vi "fit_characteristics.vi"(10 "Polynomial Coefficients":dbl[][](array[numeric]), 11 "Residue":dbl[](array[numeric])) -> (1 "Limit fail":bool[][](array[boolean]), 3 "Fit characteristics":string[][](table))   [LabVIEW 2013]
uses:
  <vilib>/Analysis/polynomials.llb/nth Derivative of Polynomial (DBL).vi
  <vilib>/Analysis/polynomials.llb/Scalar Polynomial Evaluation (DBL).vi
  <vilib>/Analysis/polynomials.llb/1D Polynomial Evaluation (DBL).vi
  <vilib>/Analysis/NI_AALPro.lvlib
panel:
  out "All x":dbl[][](array[numeric])
  out "Labels":string[](array[string])
  in  "Limits":cluster{"Min":dbl, "Max":dbl}[](array[cluster])=[{"Min"=2.0, "Max"=inf}, {"Min"=0.0, "Max"=0.3}, {"Min"=10.0, "Max"=inf}, {"Min"=10.0, "Max"=inf}, {"Min"=-inf, "Max"=-10.0}, {"Min"=10.0, "Max"=inf}, {"Min"=0.0, "Max"=1.0}]
  # "True if the corresponding  cell of the table should be highlighted as as failing limit test."
  # "Generate report of calibration results."
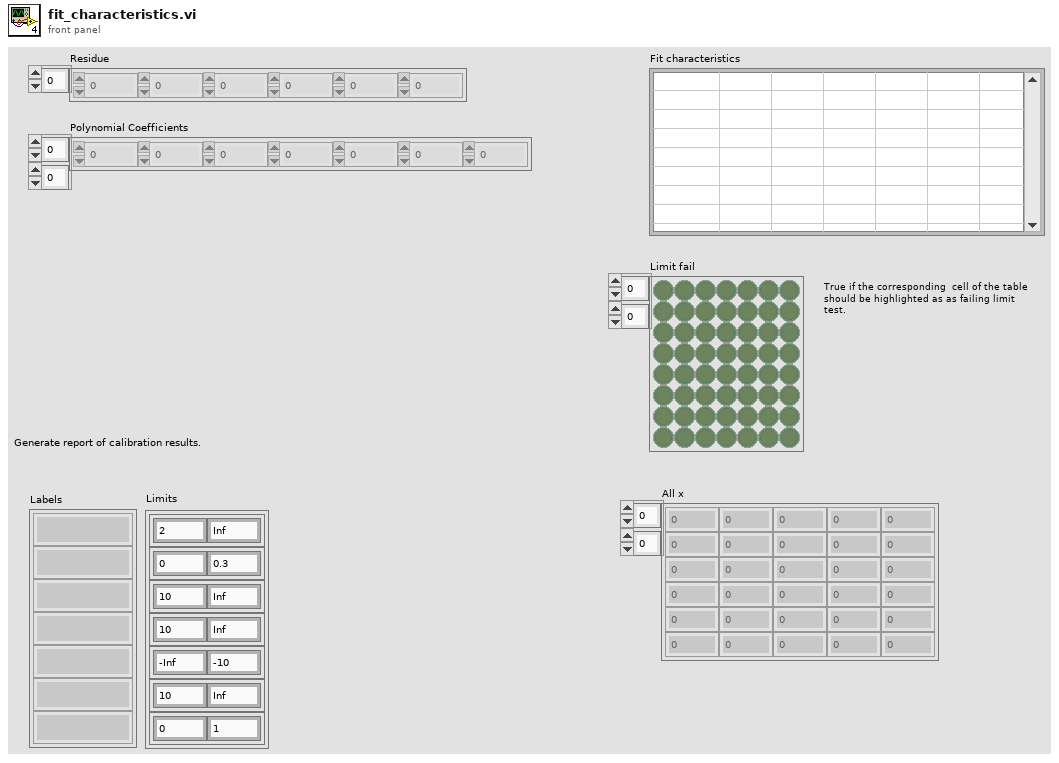
[diagram p1: front panel]
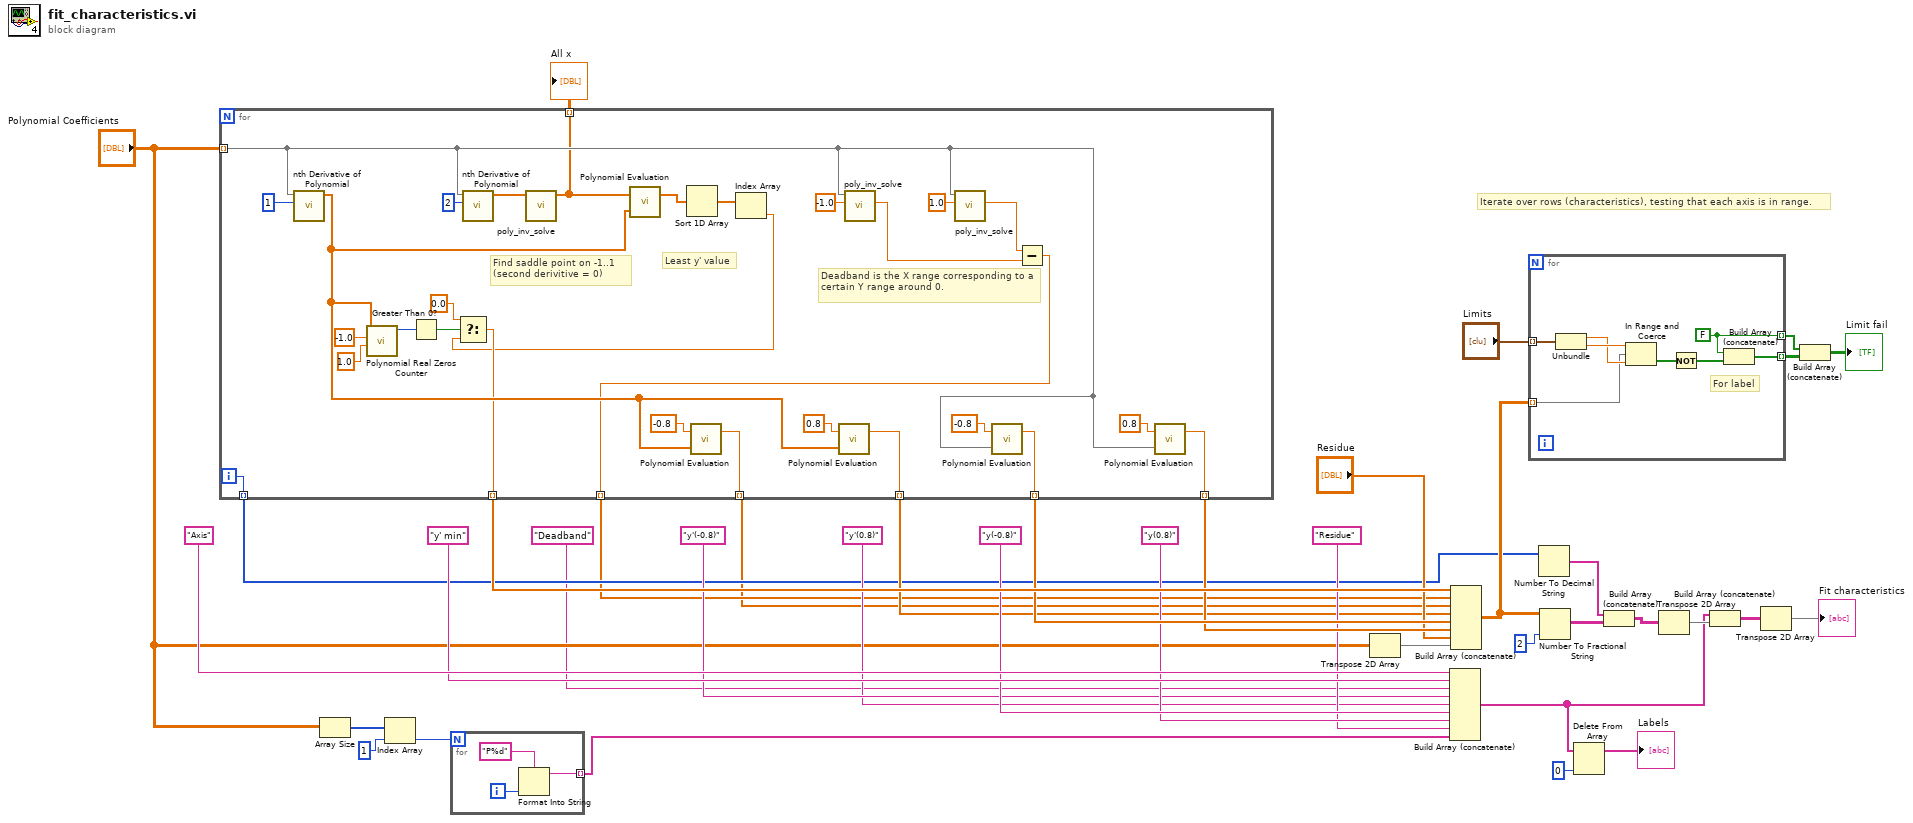
[diagram p0: block diagram]
diagram:
  # "Iterate over rows (characteristics), testing that each axis is in range."
  n1 = for {
    tunnel: "Polynomial Coefficients" -> [w46] mode=indexing
    tunnel: [w51] -> w38 mode=indexing
    tunnel: [w64] -> w37 mode=indexing
    tunnel: [w63] -> w36 mode=indexing
    tunnel: [w62] -> w11 mode=indexing
    tunnel: [w59] -> w2 mode=indexing
    tunnel: [w58] -> w28 mode=indexing
    tunnel: [w43] -> w3 mode=indexing
    tunnel: [w42] -> w1 mode=indexing
    i -> [w62]
    # "Least y' value"
    # "Deadband is the X range corresponding to a certain Y range around 0."
    # "Find saddle point on -1..1 (second derivitive = 0)"
    n2 = call-poly <vilib>:"nth Derivative of Polynomial.vi"("order"=1, "P(x)"=w46) -> ("Nth Derivative of P(x)"=w57:dbl[])  [unwired: 8 in, 1 out]
    n3 = call <vilib>:"Polynomial Real Zeros Counter.vi"("end"=1.0, "start"=-1.0, "P(x)"=w57) -> ("number of zeros"=w54:i32)  [unwired: 7 in, 1 out]
    n4 = Greater Than 0?(x=w54) -> (x > 0?=w53:bool)
    n5 = call-poly <vilib>:"nth Derivative of Polynomial.vi"("order"=2, "P(x)"=w46) -> ("Nth Derivative of P(x)"=w49:dbl[])  [unwired: 8 in, 1 out]
    n6 = call "poly_inv_solve.vi"("P(x)"=w49) -> ("All x"=w42:dbl[])  [unwired: 9 in, 1 out]
    n7 = call-poly <vilib>:"Polynomial Evaluation.vi"("P(x)"=w57, "A"=w42) -> ("P(A)"=w41:dbl[])  [unwired: 1 out]
    n8 = Sort 1D Array(array=w41) -> (sorted array=w40:dbl[])
    n9 = call-poly <vilib>:"Polynomial Evaluation.vi"("P(x)"=w57, "a"=-0.8) -> ("P(a)"=w59:dbl)  [unwired: 1 out]
    n10 = Index Array(array=w40) -> (element=w39:dbl)  [unwired: 1 in]
    n11 = Select(t=0.0, s=w53, f=w39) -> (s? t:f=w51:dbl)
    n12 = call-poly <vilib>:"Polynomial Evaluation.vi"("P(x)"=w57, "a"=0.8) -> ("P(a)"=w58:dbl)  [unwired: 1 out]
    n13 = call "poly_inv_solve.vi"("y"=-1.0, "P(x)"=w46) -> ("x"=w44:dbl)  [unwired: 8 in, 1 out]
    n14 = call "poly_inv_solve.vi"("y"=1.0, "P(x)"=w46) -> ("x"=w45:dbl)  [unwired: 8 in, 1 out]
    n15 = call-poly <vilib>:"Polynomial Evaluation.vi"("P(x)"=w46, "a"=-0.8) -> ("P(a)"=w64:dbl)  [unwired: 1 out]
    n16 = Subtract(x=w45, y=w44) -> (x-y=w43:dbl)
    n17 = call-poly <vilib>:"Polynomial Evaluation.vi"("P(x)"=w46, "a"=0.8) -> ("P(a)"=w63:dbl)  [unwired: 1 out]
  }
  "All x" <- w1
  n18 = Array Size(array="Polynomial Coefficients") -> (size(s)=w25:i32[])
  n19 = Index Array(array=w25, index=1) -> (element=w23:i32)
  n20 = for {
    N: w23 -> [_]
    tunnel: [w68] -> w22 mode=indexing
    i -> [w70]
    n21 = Format Into String(format string="P%d", w70) -> (resulting string=w68:string)  [unwired: 2 in, 1 out]
  }
  n22 = Transpose 2D Array(2D array="Polynomial Coefficients") -> (transposed array=w20:dbl[][])
  n23 = Build Array (concatenate)("Axis", "y' min", "Deadband", "y'(-0.8)", "y'(0.8)", "y(-0.8)", "y(0.8)", "Residue", w22) -> (w14:string[])
  n24 = Build Array (concatenate)(w38, w3, w2, w28, w37, w36, "Residue", w20) -> (w16:dbl[][])
  n25 = for {
    tunnel: w16 -> [w75] mode=indexing
    tunnel: "Limits" -> [w78] mode=indexing
    tunnel: [w72] -> w7 mode=indexing
    tunnel: [w71] -> w5 mode=indexing
    w71 = FALSE
    # "For label"
    n26 = Unbundle(w78) -> ("Min"=w76:dbl, "Max"=w77:dbl)
    n27 = In Range and Coerce(upper limit=w77, x=w75, lower limit=w76) -> (In Range?=w74:bool[])  [unwired: 1 out]
    n28 = Not(x=w74) -> (.not. x?=w73:bool[])
    n29 = Build Array (concatenate)(w71, w73) -> (w72:bool[])
  }
  n30 = Number To Decimal String(number=w11) -> (decimal integer string=w8:string[])  [unwired: 1 in]
  n31 = Number To Fractional String(number=w16, precision (6)=i16 2) -> (F-format string=w10:string[][])  [unwired: 2 in]
  n32 = Delete From Array(array=w14, index=0) -> (array with subset deleted=→"Labels":string[])  [unwired: 1 in, 1 out]
  n33 = Build Array (concatenate)(w8, w10) -> (w9:string[][])
  n34 = Transpose 2D Array(2D array=w9) -> (transposed array=w15:string[][])
  n35 = Build Array (concatenate)(w14, w15) -> (w19:string[][])
  n36 = Transpose 2D Array(2D array=w19) -> (transposed array=→"Fit characteristics":string[][])
  n37 = Build Array (concatenate)(w5, w7) -> (→"Limit fail":bool[][])
